vi "__Test_MemoryToLvData_NOPTR.vi"() -> ()   [LabVIEW 2019]
uses:
  __Support/LvDataToMemory_NOPTR.vi
  __Support/MemoryToLvData_NOPTR.vi
  Memory Data Access.lvlib
panel:
  out "data_Cluster":T1
  out "data_Path":path
  out "data_Str":string
  out "data_DBL":dbl
  out "data_U32":u32
  out "data_I32":i32
  out "data_Waveform":waveform(dbl)
  out "data TimeStamp":timestamp
  out "data_Bool":bool
  out "data_ArrayWav":waveform(dbl)[](array[waveform])
  out "data_ArrayDBL":dbl[](array[numeric])
  out "data_ArrayStr":string[](array[string])
  in  "Enum":T2(ring)
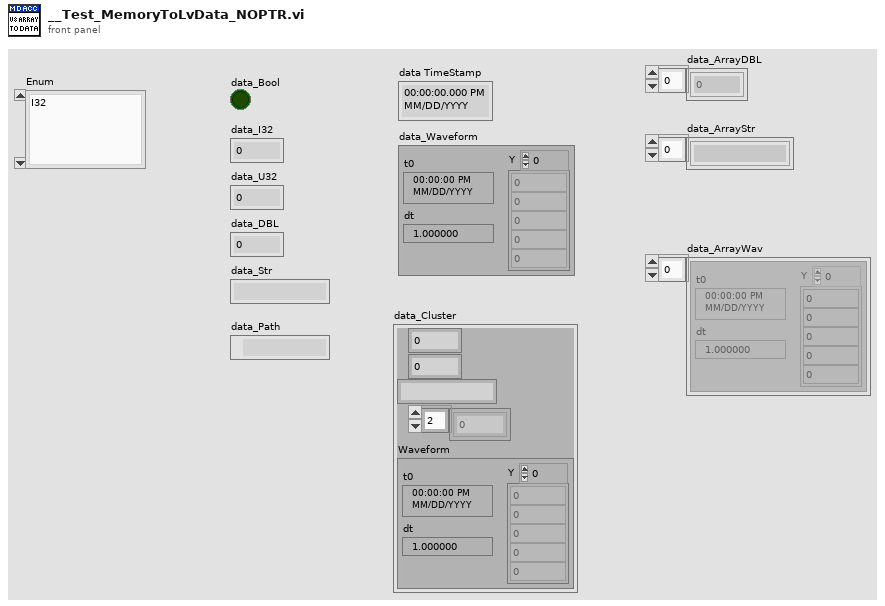
[diagram p1: front panel]
types:
  T1 = cluster{i32, dbl, string, dbl[], "Waveform":waveform(dbl)}
  T2 = enum16{"I32", "U32", "DBL", "String", "Cluster", "Array_Str", "Array_DBL", "Array_Waveform", "Bool", "TimeStamp", "Waveform", "Path"}
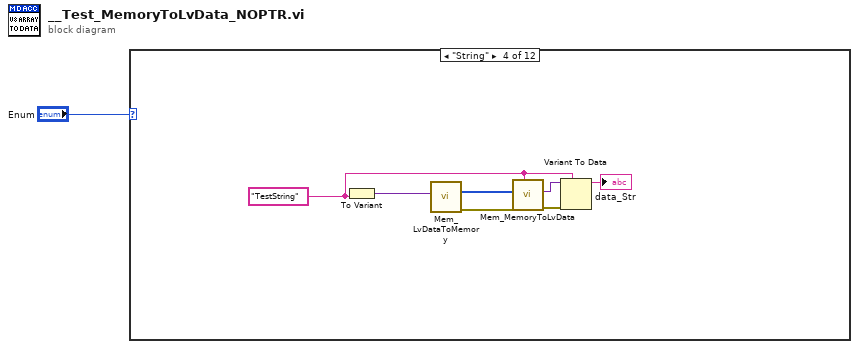
[diagram p0: block diagram]
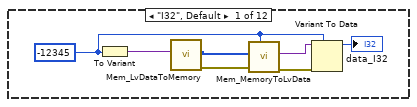
[diagram p2: hidden frame]
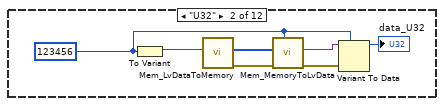
[diagram p3: hidden frame]
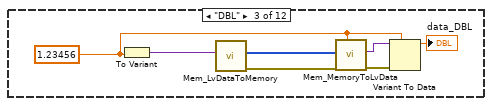
[diagram p4: hidden frame]
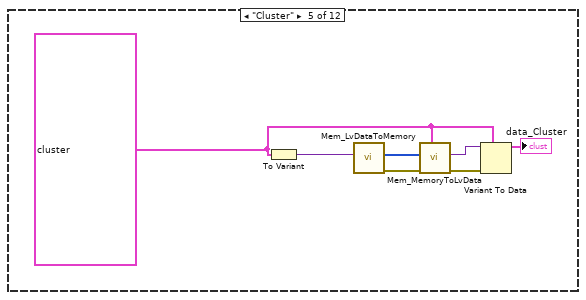
[diagram p5: hidden frame]
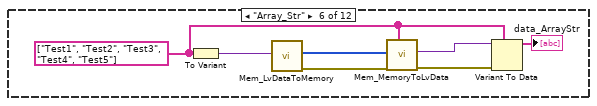
[diagram p6: hidden frame]
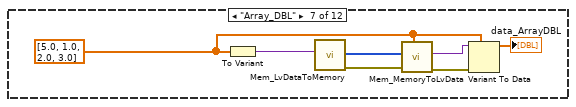
[diagram p7: hidden frame]
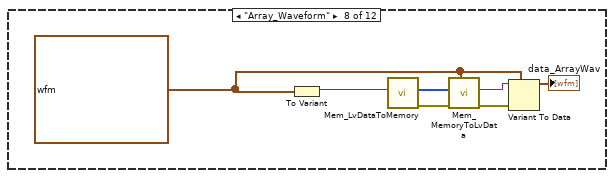
[diagram p8: hidden frame]
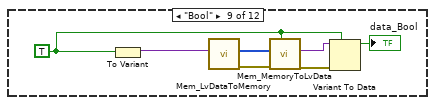
[diagram p9: hidden frame]
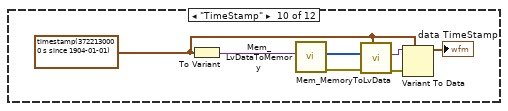
[diagram p10: hidden frame]
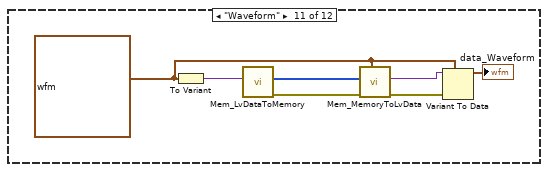
[diagram p11: hidden frame]
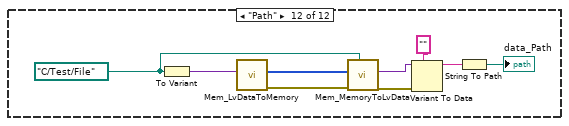
[diagram p12: hidden frame]
diagram:
  n1 = case shown="\"String\"" "Enum" {
    frame "I32", Default {
      w3 = -12345
      n2 = To Variant(anything=w3) -> (Variant=w8:variant)
      n3 = call-poly "Mem_LvDataToMemory.vi"("Payload"=w8) -> ("error out"=w6:errorcluster, "ByteArray"=w7:u8[])  [unwired: 8 in, 1 out]
      n4 = call-poly "Mem_MemoryToLvData.vi"("Type"=w3, "error in (no error)"=w6, "ByteArray"=w7) -> ("error out"=w5:errorcluster, "data"=w4:variant)  [unwired: 5 in, 2 out]
      n5 = Variant To Data(error in=w5, type=w3, Variant=w4) -> (data=→"data_I32":i32)  [unwired: 1 out]
    }
    frame "U32" {
      w10 = u32 123456
      n6 = To Variant(anything=w10) -> (Variant=w15:variant)
      n7 = call-poly "Mem_LvDataToMemory.vi"("Payload"=w15) -> ("error out"=w13:errorcluster, "ByteArray"=w14:u8[])  [unwired: 8 in, 1 out]
      n8 = call-poly "Mem_MemoryToLvData.vi"("Type"=w10, "error in (no error)"=w13, "ByteArray"=w14) -> ("error out"=w11:errorcluster, "data"=w12:variant)  [unwired: 5 in, 2 out]
      n9 = Variant To Data(error in=w11, type=w10, Variant=w12) -> (data=→"data_U32":u32)  [unwired: 1 out]
    }
    frame "DBL" {
      w17 = 1.23456
      n10 = To Variant(anything=w17) -> (Variant=w22:variant)
      n11 = call-poly "Mem_LvDataToMemory.vi"("Payload"=w22) -> ("error out"=w20:errorcluster, "ByteArray"=w21:u8[])  [unwired: 8 in, 1 out]
      n12 = call-poly "Mem_MemoryToLvData.vi"("Type"=w17, "error in (no error)"=w20, "ByteArray"=w21) -> ("error out"=w19:errorcluster, "data"=w18:variant)  [unwired: 5 in, 2 out]
      n13 = Variant To Data(error in=w19, type=w17, Variant=w18) -> (data=→"data_DBL":dbl)  [unwired: 1 out]
    }
    frame "String" {
      w24 = "TestString"
      n14 = To Variant(anything=w24) -> (Variant=w29:variant)
      n15 = call-poly "Mem_LvDataToMemory.vi"("Payload"=w29) -> ("error out"=w27:errorcluster, "ByteArray"=w28:u8[])  [unwired: 8 in, 1 out]
      n16 = call-poly "Mem_MemoryToLvData.vi"("Type"=w24, "error in (no error)"=w27, "ByteArray"=w28) -> ("error out"=w26:errorcluster, "data"=w25:variant)  [unwired: 5 in, 2 out]
      n17 = Variant To Data(error in=w26, type=w24, Variant=w25) -> (data=→"data_Str":string)  [unwired: 1 out]
    }
    frame "Cluster" {
      w31 = T1 {1245, 1.2345, "TestString", [0.0, 1.0, 2.0, 3.0], "Waveform"={"t0"=timestamp(3722126400 s since 1904-01-01), "dt"=1.0, "Y"=[1.0, 2.0, 3.0, 4.0]}}
      n18 = To Variant(anything=w31) -> (Variant=w36:variant)
      n19 = call-poly "Mem_LvDataToMemory.vi"("Payload"=w36) -> ("error out"=w33:errorcluster, "ByteArray"=w35:u8[])  [unwired: 8 in, 1 out]
      n20 = call-poly "Mem_MemoryToLvData.vi"("Type"=w31, "error in (no error)"=w33, "ByteArray"=w35) -> ("error out"=w32:errorcluster, "data"=w34:variant)  [unwired: 5 in, 2 out]
      n21 = Variant To Data(error in=w32, type=w31, Variant=w34) -> (data=→"data_Cluster":T1)  [unwired: 1 out]
    }
    frame "Array_Str" {
      w40 = string[] ["Test1", "Test2", "Test3", "Test4", "Test5"]
      n22 = To Variant(anything=w40) -> (Variant=w43:variant)
      n23 = call-poly "Mem_LvDataToMemory.vi"("Payload"=w43) -> ("error out"=w38:errorcluster, "ByteArray"=w42:u8[])  [unwired: 8 in, 1 out]
      n24 = call-poly "Mem_MemoryToLvData.vi"("Type"=w40, "error in (no error)"=w38, "ByteArray"=w42) -> ("error out"=w37:errorcluster, "data"=w41:variant)  [unwired: 5 in, 2 out]
      n25 = Variant To Data(error in=w37, type=w40, Variant=w41) -> (data=→"data_ArrayStr":string[])  [unwired: 1 out]
    }
    frame "Array_DBL" {
      w45 = dbl[] [5.0, 1.0, 2.0, 3.0]
      n26 = To Variant(anything=w45) -> (Variant=w50:variant)
      n27 = call-poly "Mem_LvDataToMemory.vi"("Payload"=w50) -> ("error out"=w48:errorcluster, "ByteArray"=w49:u8[])  [unwired: 8 in, 1 out]
      n28 = call-poly "Mem_MemoryToLvData.vi"("Type"=w45, "error in (no error)"=w48, "ByteArray"=w49) -> ("error out"=w46:errorcluster, "data"=w47:variant)  [unwired: 5 in, 2 out]
      n29 = Variant To Data(error in=w46, type=w45, Variant=w47) -> (data=→"data_ArrayDBL":dbl[])  [unwired: 1 out]
    }
    frame "Array_Waveform" {
      w52 = waveform(dbl)[] [{"t0"=timestamp(3705278400 s since 1904-01-01), "dt"=1.0, "Y"=[1.0, 2.0, 3.0]}, {"t0"=timestamp(3705278400 s since 1904-01-01), "dt"=1.0, "Y"=[4.0, 5.0, 6.0]}]
      n30 = To Variant(anything=w52) -> (Variant=w57:variant)
      n31 = call-poly "Mem_LvDataToMemory.vi"("Payload"=w57) -> ("error out"=w54:errorcluster, "ByteArray"=w56:u8[])  [unwired: 8 in, 1 out]
      n32 = call-poly "Mem_MemoryToLvData.vi"("Type"=w52, "error in (no error)"=w54, "ByteArray"=w56) -> ("error out"=w55:errorcluster, "data"=w53:variant)  [unwired: 5 in, 2 out]
      n33 = Variant To Data(error in=w55, type=w52, Variant=w53) -> (data=→"data_ArrayWav":waveform(dbl)[])  [unwired: 1 out]
    }
    frame "Bool" {
      w59 = TRUE
      n34 = To Variant(anything=w59) -> (Variant=w64:variant)
      n35 = call-poly "Mem_LvDataToMemory.vi"("Payload"=w64) -> ("error out"=w60:errorcluster, "ByteArray"=w63:u8[])  [unwired: 8 in, 1 out]
      n36 = call-poly "Mem_MemoryToLvData.vi"("Type"=w59, "error in (no error)"=w60, "ByteArray"=w63) -> ("error out"=w61:errorcluster, "data"=w62:variant)  [unwired: 5 in, 2 out]
      n37 = Variant To Data(error in=w61, type=w59, Variant=w62) -> (data=→"data_Bool":bool)  [unwired: 1 out]
    }
    frame "TimeStamp" {
      w66 = timestamp(3722130000 s since 1904-01-01)
      n38 = To Variant(anything=w66) -> (Variant=w71:variant)
      n39 = call-poly "Mem_LvDataToMemory.vi"("Payload"=w71) -> ("error out"=w69:errorcluster, "ByteArray"=w70:u8[])  [unwired: 8 in, 1 out]
      n40 = call-poly "Mem_MemoryToLvData.vi"("Type"=w66, "error in (no error)"=w69, "ByteArray"=w70) -> ("error out"=w68:errorcluster, "data"=w67:variant)  [unwired: 5 in, 2 out]
      n41 = Variant To Data(error in=w68, type=w66, Variant=w67) -> (data=→"data TimeStamp":timestamp)  [unwired: 1 out]
    }
    frame "Waveform" {
      w73 = waveform(dbl) {"t0"=timestamp(3722126400 s since 1904-01-01), "dt"=1.0, "Y"=[1.0, 2.0, 3.0, 4.0]} ("Waveform")
      n42 = To Variant(anything=w73) -> (Variant=w78:variant)
      n43 = call-poly "Mem_LvDataToMemory.vi"("Payload"=w78) -> ("error out"=w76:errorcluster, "ByteArray"=w77:u8[])  [unwired: 8 in, 1 out]
      n44 = call-poly "Mem_MemoryToLvData.vi"("Type"=w73, "error in (no error)"=w76, "ByteArray"=w77) -> ("error out"=w74:errorcluster, "data"=w75:variant)  [unwired: 5 in, 2 out]
      n45 = Variant To Data(error in=w74, type=w73, Variant=w75) -> (data=→"data_Waveform":waveform(dbl))  [unwired: 1 out]
    }
    frame "Path" {
      w82 = path "C:/Test/File"
      n46 = To Variant(anything=w82) -> (Variant=w87:variant)
      n47 = call-poly "Mem_LvDataToMemory.vi"("Payload"=w87) -> ("error out"=w85:errorcluster, "ByteArray"=w86:u8[])  [unwired: 8 in, 1 out]
      n48 = call-poly "Mem_MemoryToLvData.vi"("Type"=w82, "error in (no error)"=w85, "ByteArray"=w86) -> ("error out"=w84:errorcluster, "data"=w83:variant)  [unwired: 5 in, 2 out]
      n49 = Variant To Data(error in=w84, type="", Variant=w83) -> (data=w80:string)  [unwired: 1 out]
      n50 = String To Path(string=w80) -> (path=→"data_Path":path)
    }
  }
